vi "Starting.vi"(4 "Async Elements":refnum<class "Async Elements.lvclass">, 6 "VI Ref":refnum<vi>, 7 "Actor in":refnum<class "Actor.lvclass">, 9 "Transport":refnum<class "Transport.lvclass">) -> (0 "Error out":errorcluster, 5 "Actor out":refnum<class "Actor.lvclass">)   [LabVIEW 2020, in "jettl.lvlib"]
uses:
  jettl.lvlib
  Actor/Actor.lvclass
  Transport/Transport.lvclass
  Async Elements/Async Elements.lvclass
  Base Async Elements/Base Async Elements/Base Async Elements.lvclass/Base Async Elements.ctl
  Async Elements.ctl
  Attributes/Attributes.lvclass
  Base Attributes/Base Attributes/Base Attributes.lvclass/Base Attributes.ctl
  Teardown Location.ctl
  Base Attributes/Init Attributes.vi
  Base Attributes/Base Attributes/Init Attributes.vi
  Base Attributes/Base Attributes/Base Attributes.lvclass
  C:/git/jettl/src/jettl/jettl/Attributes/Attributes.lvclass
  Base Async Elements/Base Async Elements/Base Async Elements.lvclass
  Msg/Msg.lvclass
  Base Async Elements/Base Async Elements.lvlib
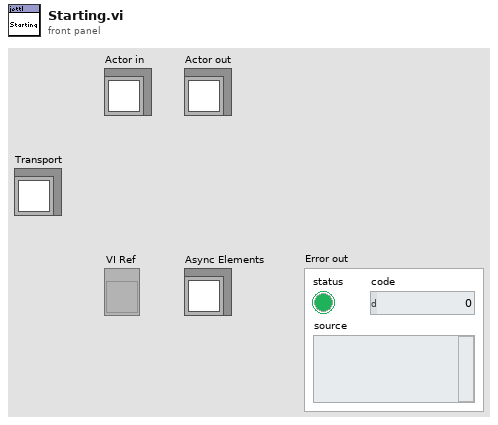
[diagram p1: front panel]
types:
  T1 = typedef "jettl.lvlib/Async Elements.ctl" = cluster{"Attributes":refnum<class "Attributes.lvclass">, "Error":errorcluster}
  T2 = typedef "jettl.lvlib/Teardown Location.ctl" = enum16{"Starting", "Should Stop"}
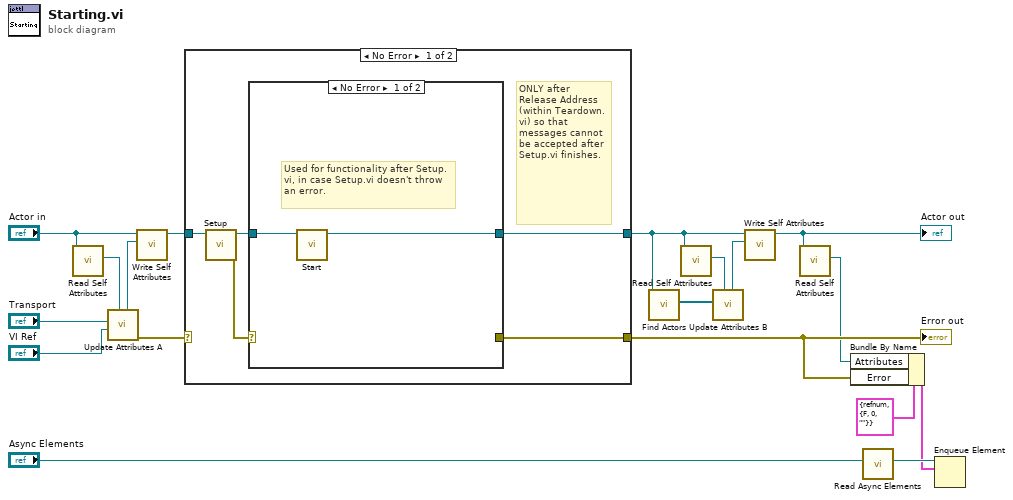
[diagram p0: block diagram]
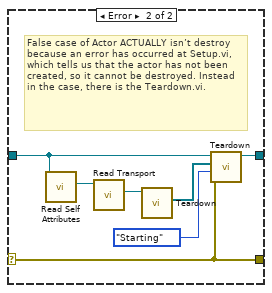
[diagram p2: hidden frame]
diagram:
  n1 = call-dynamic "Read Self Attributes.vi"("Actor in"="Actor in") -> ("Self Attributes"=w3:refnum<class "Attributes.lvclass">)  [unwired: 10 in]
  n2 = call "Update Attributes A.vi"("Attributes in"=w3, "VI Ref"="VI Ref", "Transport"="Transport") -> ("Error out"=w18:errorcluster, "Attributes out"=w14:refnum<class "Attributes.lvclass">)  [unwired: 7 in]
  n3 = call-dynamic "Write Self Attributes.vi"("Self Attributes"=w14, "Actor in"="Actor in") -> ("Actor out"=w15:refnum<class "Actor.lvclass">)  [unwired: 9 in]
  n4 = case shown="No Error" w18 {
    selector: w18 -> [_ w34]
    tunnel: w15 -> [w20 w33]
    tunnel: [w21 w33] -> w9
    tunnel: [w19 w34] -> w17
    frame No Error {
      # "ONLY after Release Address (within Teardown.vi) so that messages cannot be accepted after Setup.vi finishes."
      n5 = call-dynamic "Setup.vi"("Actor in"=w20) -> ("Error out"=w22:errorcluster, "Actor out"=w23:refnum<class "Actor.lvclass">)  [unwired: 9 in]
      n6 = case shown="No Error" w22 {
        selector: w22 -> [_ w31]
        tunnel: w23 -> [w25 w28]
        tunnel: [_ w31] -> w19
        tunnel: [w24 w32] -> w21
        frame No Error {
          # "Used for functionality after Setup.vi, in case Setup.vi doesn't throw an error."
          n7 = call-dynamic "Start.vi"("Actor in"=w25) -> ("Actor out"=w24:refnum<class "Actor.lvclass">)  [unwired: 10 in]
        }
        frame Error {
          # "False case of Actor ACTUALLY isn’t destroy because an error has occurred at Setup.vi, which tells us that the actor has not been created, so it cannot be destroyed. Instead in the case, there is the Teardown.vi."
          n8 = call-dynamic "Read Self Attributes.vi"("Actor in"=w28) -> ("Self Attributes"=w27:refnum<class "Attributes.lvclass">)  [unwired: 10 in]
          n9 = call-dynamic "Read Transport.vi"("Attributes in"=w27) -> ("Transport"=w26:refnum<class "Transport.lvclass">)  [unwired: 10 in]
          n10 = call-dynamic "Teardown.vi"("Transport in"=w26) -> ("Unheard Msgs"=w29:refnum<class "Msg.lvclass">[])  [unwired: 10 in]
          n11 = call-dynamic "Teardown.vi"("Error in"=w31, "Teardown Location"=Teardown_Location."Starting", "Unheard Msgs"=w29, "Actor in"=w28) -> ("Actor out"=w32:refnum<class "Actor.lvclass">)  [unwired: 7 in]
        }
      }
    }
    frame Error {
    }
  }
  "Error out" <- w17
  n12 = call-dynamic "Find Actors.vi"("Actor in"=w9) -> ("Actors"=w8:refnum<class "Actor.lvclass">[])  [unwired: 10 in]
  n13 = call-dynamic "Read Self Attributes.vi"("Actor in"=w9) -> ("Self Attributes"=w12:refnum<class "Attributes.lvclass">)  [unwired: 10 in]
  n14 = call "Update Attributes B.vi"("Attributes in"=w12, "Actors"=w8) -> ("Attributes out"=w11:refnum<class "Attributes.lvclass">)  [unwired: 9 in]
  n15 = call-dynamic "Write Self Attributes.vi"("Self Attributes"=w11, "Actor in"=w9) -> ("Actor out"=w10:refnum<class "Actor.lvclass">)  [unwired: 9 in]
  "Actor out" <- w10
  n16 = call-dynamic "Read Self Attributes.vi"("Actor in"=w10) -> ("Self Attributes"=w16:refnum<class "Attributes.lvclass">)  [unwired: 10 in]
  n17 = Bundle By Name(cluster=T1 {"Attributes"=refnum, "Error"={"status"=FALSE, "code"=0, "source"=""}} ("element"), "Attributes"=w16, "Error"=w17) -> (w5:T1)
  n18 = call "Read Async Elements.vi"("Async Elements"="Async Elements") -> ("Async Elements"=w6:refnum<queue>)  [unwired: 10 in]
  n19 = Enqueue Element(queue=w6, element=w5) -> ()  [unwired: 2 in, 3 out]
